vi "Additional_Post_Process_SJ_Data.vi"() -> ()   [LabVIEW 2012]
uses:
  Process_States.ctl
  Controls/SJ_Test_Matrix.ctl
  Controls/Analysis_info_cluster.ctl
  Controls/Inst_type.ctl
  Controls/Instrument_Array.ctl
  <vilib>/gmath/NumericalOptimization/stopping criteria.ctl
  <vilib>/Analysis/baseanly.llb/Scale 1D.vi
  <vilib>/Analysis/NI_AALBase.lvlib
  <vilib>/gmath/NI_Gmath.lvlib
panel:
  out "New Filename":path
  out "Prog bar":sgl(slide) scale=0.0..1.0
  out "Message":string
  in  "Max Iterations":i32=3000
  in  "Tolerance":dbl=0.0001
  in  "Raw Data Folder":path=path "F:/Enflo_Data_Local/2011/Aero_Tunnel/nick_martin/Raw_Measurements/11-2011/New_SJ_TestI_xls"
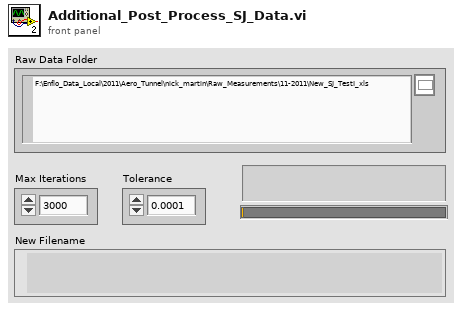
[diagram p1: front panel]
types:
  T1 = typedef "Process_States.ctl" = enum16{"Load Data", "Fit Parabolas", "Save Data"}
  T2 = typedef "SJ_Test_Matrix.ctl" = cluster{"Channel Data":cluster{"Amplitude (V)":dbl, "Phase Average":dbl[][], "Phase Angle":dbl[], "Frequency (Hz)":dbl, "AS Freq":dbl, "Zero":dbl, "Analysis info cluster":T3, "Radius":dbl[], "Beta":dbl, "Phi":dbl, "|Qd|":dbl, "Qd":dbl[]}[]}
  T3 = typedef "Analysis_info_cluster.ctl" = cluster{"Colour":u32, "Inst type":T4, "Inst name":string, "Symbol":string, "Code name":string, "Extra Info":string, "Inst Array":T5, "Extra Titles":string[], "Extra Values":string[], "U":dbl, "u^2":dbl, "u^3":dbl, "u^4":dbl, "Skew_u":dbl, "Kurt_u":dbl, "Sd Error in Mean":dbl, "% u'/U":dbl, "X":dbl, "Y":dbl, "Z":dbl, "Timescale integral to 25%":dbl, "Sd Error in Variance":dbl, "Calib File":path, "Calib Constants":dbl[], "Output Position":bool, "Full Stats":bool, "Av Sampling Rate":dbl, "Av No of Samples":dbl, "Total Meas Time (s)":dbl, "ADAM Ch Name":string}
  T4 = typedef "Inst_type.ctl" = enum16{"Propeller anemometer", "Raw voltage", "Pressure Transducer", "Pitot-static tube", "Preston tube", "Hot wire", "Cross wire 1", "Cross wire 2", "Generic Linear", "Generic Polynomial", "Generic BackPoly", "Fast FID", "Thermocouple", "Cold wire", "Pulsed Wire", "LDA Vel", "LDA Tran time", "LDA Arr time"}
  T5 = typedef "Instrument_Array.ctl" = enum16{"PWA", "LDA", "Analogue"}
  T6 = typedef "NI_Gmath.lvlib/stopping criteria.ctl" = cluster{"function tolerance":dbl, "parameter tolerance":dbl, "max iterations":i32, "max function calls":i32, "gradient tolerance":dbl, "max time (sec)":dbl}
  T7 = cluster{"Amplitude (V)":dbl, "Phase Average":dbl[][], "Phase Angle":dbl[], "Frequency (Hz)":dbl, "AS Freq":dbl, "Zero":dbl, "Analysis info cluster":T3, "Radius":dbl[], "Beta":dbl, "Phi":dbl, "|Qd|":dbl, "Qd":dbl[]}[]
  T8 = cluster{"Amplitude (V)":dbl, "Phase Average":dbl[][], "Phase Angle":dbl[], "Frequency (Hz)":dbl, "AS Freq":dbl, "Zero":dbl, "Analysis info cluster":T3, "Radius":dbl[], "Beta":dbl, "Phi":dbl, "|Qd|":dbl, "Qd":dbl[]}
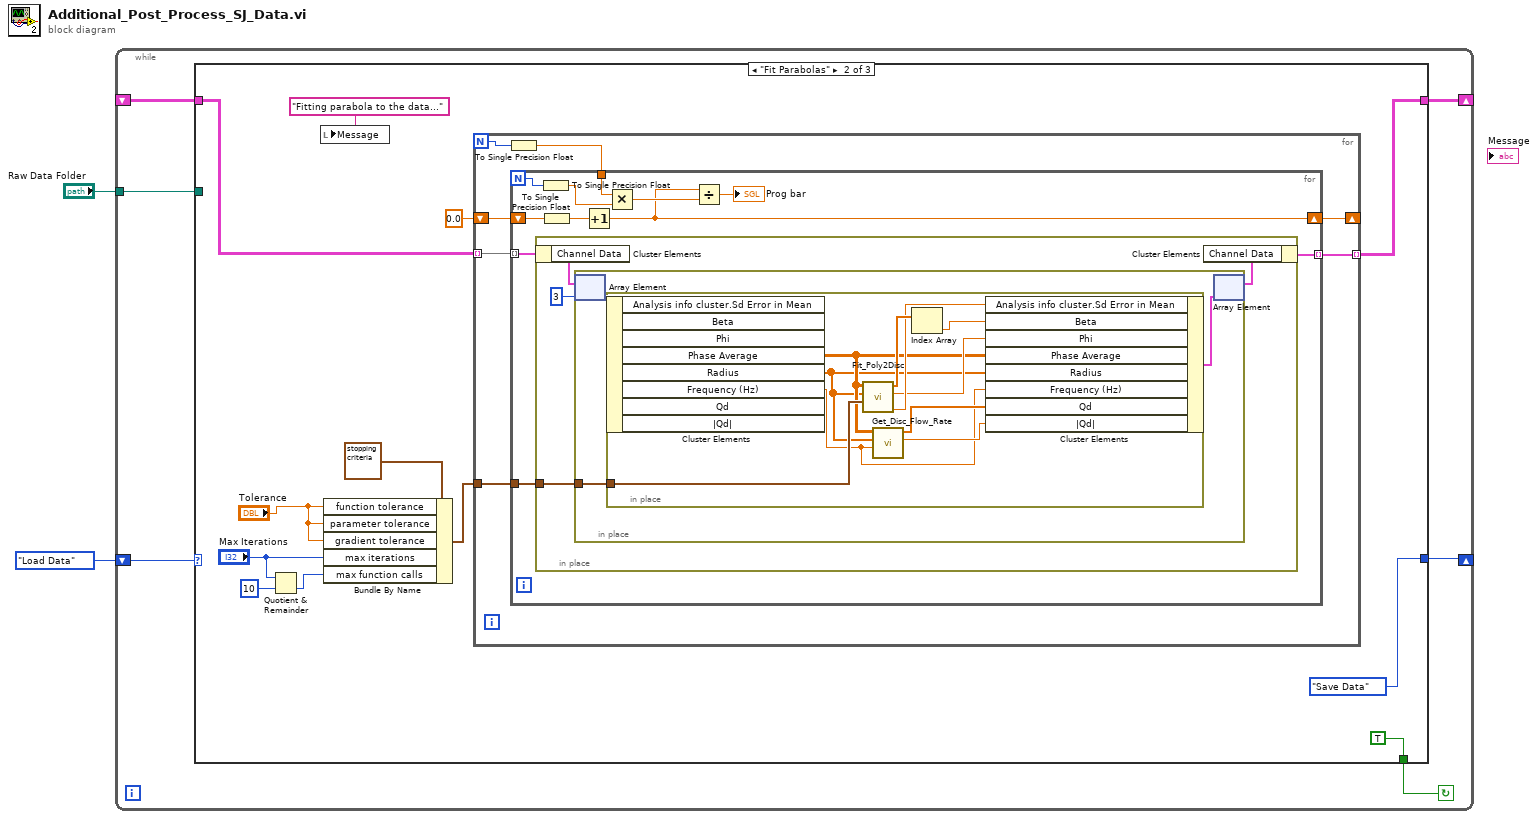
[diagram p0: block diagram]
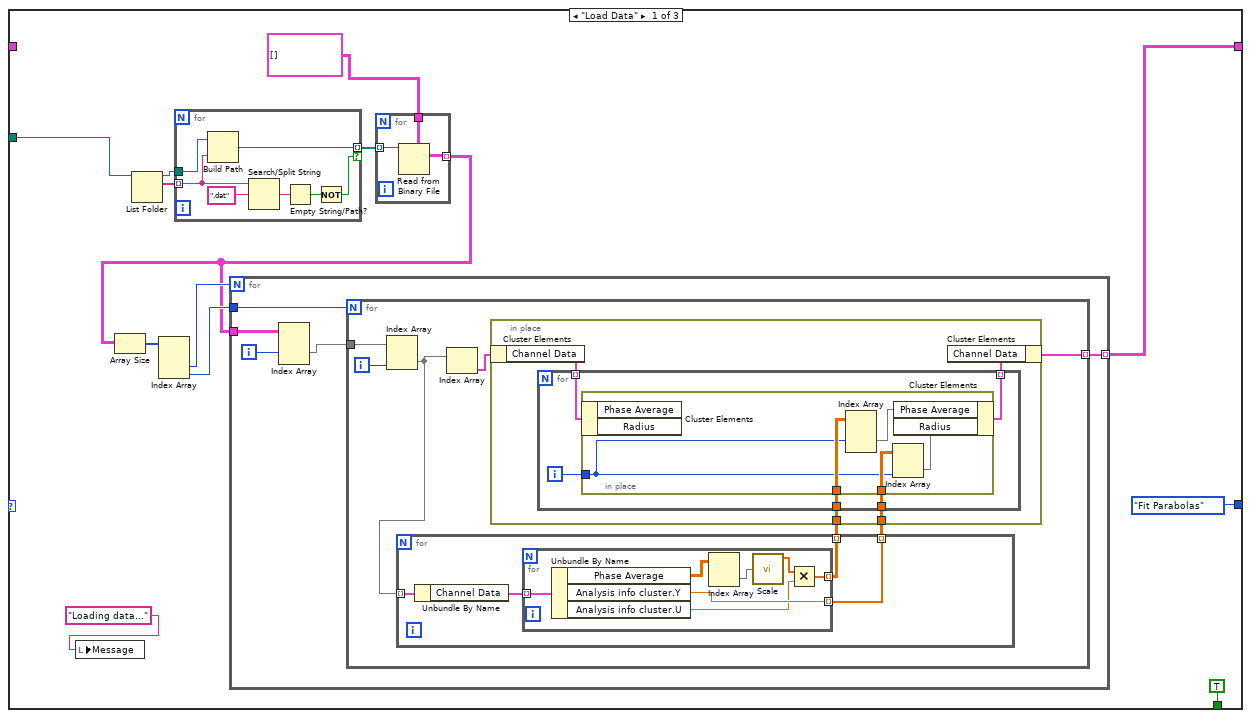
[diagram p2: hidden frame]
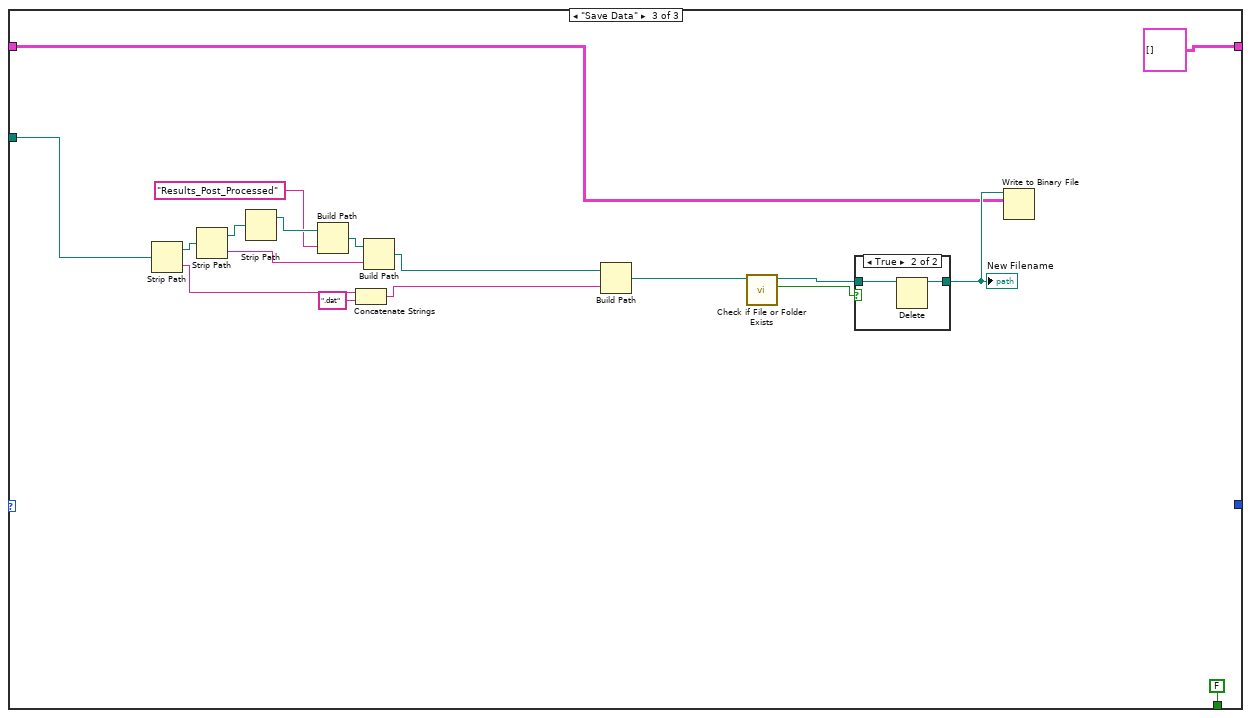
[diagram p3: hidden frame]
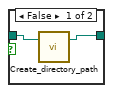
[diagram p4: hidden frame]
diagram:
  n1 = while {
    shift-right: [w7] -> _
    shift-left: _ -> [w6]
    shift-right: [w5] -> _
    shift-left: Process_States."Load Data" -> [w8]
    tunnel: "Raw Data Folder" -> [w3]
    stop <- w4 continue-if-true
    n2 = case shown="\"Fit Parabolas\"" w8 {
      tunnel: [w18 w71 T2[][] []] -> w7
      tunnel: w6 -> [_ w72 w116]
      tunnel: [Process_States."Fit Parabolas" ("Enum") Process_States."Save Data" ("Enum") _] -> w5
      tunnel: [TRUE TRUE FALSE] -> w4
      tunnel: w3 -> [w10 _ w120]
      frame "Load Data" {
        n3 = local write "Message"("Loading data..." ("Message")) -> ()
        n4 = List Folder(path=w10) -> (path out=w13:path, filenames=w12:string[])  [unwired: 3 in, 2 out]
        n5 = for {
          tunnel: w12 -> [w26] mode=indexing
          tunnel: [w25] -> w14 mode=indexing if=w29
          tunnel: w13 -> [w27]
          n6 = Build Path(base path=w27, name or relative path=w26) -> (appended path=w25:path)
          n7 = Search/Split String(string=w26, search string/char (-)=".dat" ("regular expression")) -> (match + rest of string=w28:string)  [unwired: 1 in, 2 out]
          n8 = Empty String/Path?(string/path=w28) -> (empty?=w30:bool)
          n9 = Not(x=w30) -> (.not. x?=w29:bool)
        }
        n10 = for {
          tunnel: w14 -> [w24] mode=indexing
          tunnel: T2[][] [] -> [w23]
          tunnel: [w22] -> w11 mode=indexing
          n11 = Read from Binary File(5:w23, 11:w24) -> (2:w22:T2[][])  [unwired: 4 in, 3 out]
        }
        n12 = Array Size(array=w11) -> (size(s)=w21:i32[])
        n13 = Index Array(array=w21) -> (element #2=w20:i32, element #3=w19:i32)  [unwired: 3 in, 1 out]
        n14 = for {
          N: w20 -> [_]
          tunnel: w11 -> [w36]
          tunnel: w19 -> [w33]
          tunnel: [w32] -> w18 mode=indexing
          i -> [w35]
          n15 = Index Array(array=w36, index (dim 1)=w35) -> (element=w34:T2[][])  [unwired: 2 in]
          n16 = for {
            N: w33 -> [_]
            tunnel: w34 -> [w43]
            tunnel: [w37] -> w32 mode=indexing
            i -> [w42]
            n17 = Index Array(array=w43, index (col)=w42) -> (element=w41:T2[])  [unwired: 1 in]
            n18 = for {
              tunnel: w41 -> [w61] mode=indexing
              tunnel: [w58] -> w39 mode=indexing
              tunnel: [w59] -> w38 mode=indexing
              n19 = Unbundle By Name(w61) -> ("Channel Data"=w60:T7)
              n20 = for {
                tunnel: [w68] -> w59 mode=indexing
                tunnel: [w62] -> w58 mode=indexing
                tunnel: w60 -> [w65] mode=indexing
                n21 = Unbundle By Name(w65) -> ("Phase Average"=w67:dbl[][], "Analysis info cluster.Y"=w68:dbl, "Analysis info cluster.U"=w63:dbl)
                n22 = Index Array(array=w67) -> (element=w66:dbl[])  [unwired: 2 in]
                n23 = call-poly <vilib>:"Scale.vi"("X"=w66) -> ("Y=(X-offset)/scale"=w64:dbl[])  [unwired: 3 out]
                n24 = Multiply(x=w64, y=w63) -> (x*y=w62:dbl[])
              }
            }
            n25 = Index Array(array=w41) -> (element=w40:T2)  [unwired: 1 in]
            n26 = in-place {
              in-place-border: w39 -> [w47]
              in-place-border: w38 -> [w46]
              n27 = in-place-cluster #1(w40) -> ("Channel Data"=w44:T7)
              n28 = for {
                tunnel: w47 -> [w49]
                tunnel: w46 -> [w48]
                tunnel: [w52] -> w45 mode=indexing
                tunnel: w44 -> [w51] mode=indexing
                i -> [w50]
                n29 = in-place {
                  in-place-border: w49 -> [w57]
                  in-place-border: w50 -> [w54]
                  in-place-border: w48 -> [w55]
                  n30 = in-place-cluster #2(w51) -> ()  [unwired: 2 out]
                  n31 = Index Array(array=w57, index (dim 1)=w54) -> (element=w56:dbl[][])  [unwired: 2 in]
                  n32 = Index Array(array=w55, index (col)=w54) -> (element=w53:dbl[])  [unwired: 1 in]
                  n33 = in-place-cluster #2("Phase Average"=w56, "Radius"=w53) -> (w52:T8)
                }
              }
              n34 = in-place-cluster #1("Channel Data"=w45) -> (w37:T2)
            }
          }
        }
      }
      frame "Fit Parabolas" {
        n35 = Quotient & Remainder(x="Max Iterations", y=10) -> (floor(x/y)=w74:i32)  [unwired: 1 out]
        n36 = local write "Message"("Fitting parabola to the data..." ("Message")) -> ()
        n37 = Bundle By Name(cluster=T6 {"function tolerance"=0.001, "parameter tolerance"=0.001, "max iterations"=100, "max function calls"=1000, "gradient tolerance"=0.001, "max time (sec)"=-1.0} ("stopping criteria"), "function tolerance"="Tolerance", "parameter tolerance"="Tolerance", "gradient tolerance"="Tolerance", "max iterations"="Max Iterations", "max function calls"=w74) -> (w77:T6)
        n38 = for {
          N -> [w85]
          tunnel: w72 -> [w87] mode=indexing
          tunnel: w77 -> [w86]
          tunnel: [w84] -> w71 mode=indexing
          shift-right: [w81] -> _
          shift-left: sgl 0.0 ("single precision float") -> [w82]
          n39 = To Single Precision Float(number=w85) -> (single precision float=w83:sgl)
          n40 = for {
            N -> [w96]
            tunnel: w87 -> [w98] mode=indexing
            tunnel: w86 -> [w97]
            tunnel: w83 -> [w94]
            tunnel: [w92] -> w84 mode=indexing
            shift-right: [w88] -> w81
            shift-left: w82 -> [w90]
            n41 = in-place {
              in-place-border: w97 -> [w99]
              n42 = in-place-cluster #3(w98) -> ("Channel Data"=w102:T7)
              n43 = in-place {
                in-place-border: w99 -> [w104]
                n44 = in-place-array #4(w102, 3) -> (w105:T8)
                n45 = in-place {
                  in-place-border: w104 -> [w115]
                  n46 = in-place-cluster #5(w105) -> ("Phase Average"=w110:dbl[][], "Radius"=w109:dbl[], "Frequency (Hz)"=w106:dbl)  [unwired: 5 out]
                  n47 = call "Fit_Poly2Disc.vi"("stopping criteria"=w115, "Rc"=w109, "Xd(t,r)"=w110) -> ("f(minimum)"=w112:dbl, "Sine Phase"=w111:dbl, "P(x)"=w114:dbl[])  [unwired: 5 in, 1 out]
                  n48 = call "Get_Disc_Flow_Rate.vi"("Jet Frequency"=w106, "Radius"=w109, "Phase Average"=w110) -> ("|Qd|"=w107:dbl, "Qd(t)"=w108:dbl[])  [unwired: 6 in, 1 out]
                  n49 = Index Array(array=w114) -> (element=w113:dbl)  [unwired: 1 in]
                  n50 = in-place-cluster #5("Analysis info cluster.Sd Error in Mean"=w112, "Beta"=w113, "Phi"=w111, "Phase Average"=w110, "Radius"=w109, "Frequency (Hz)"=w106, "Qd"=w108, "|Qd|"=w107) -> (w103:T8)
                }
                n51 = in-place-array #4(w103) -> (w100:T7)  [unwired: 1 out]
              }
              n52 = in-place-cluster #3("Channel Data"=w100) -> (w92:T2)
            }
            n53 = To Single Precision Float(number=w96) -> (single precision float=w95:sgl)
            n54 = To Single Precision Float(number=w90) -> (single precision float=w89:sgl)
            n55 = Increment(x=w89) -> (x+1=w88:sgl)
            n56 = Multiply(x=w94, y=w95) -> (x*y=w93:sgl)
            n57 = Divide(x=w88, y=w93) -> (x/y=→"Prog bar":sgl)
          }
        }
      }
      frame "Save Data" {
        n58 = Strip Path(path=w120) -> (stripped path=w128:path, name=w119:string)
        n59 = Strip Path(path=w128) -> (stripped path=w127:path, name=w123:string)
        n60 = Strip Path(path=w127) -> (stripped path=w126:path)  [unwired: 1 out]
        n61 = Build Path(base path=w126, name or relative path="Results_Post_Processed") -> (appended path=w124:path)
        n62 = Concatenate Strings(w119, ".dat" ("string")) -> (w117:string)
        n63 = Build Path(base path=w124, name or relative path=w123) -> (appended path=w122:path)
        n64 = Build Path(base path=w122, name or relative path=w117) -> (appended path=w121:path)
        n65 = call <vilib>:"Check if File or Folder Exists.vi"("path"=w121) -> ("file or folder exists?"=w131:bool, "dup path"=w130:path)  [unwired: 8 in, 1 out]
        n66 = case shown="True" w131 {
          tunnel: w130 -> [w135 w137]
          tunnel: [w134 w136] -> w129
          frame False {
            n67 = call "Create_directory_path.vi"("Path name"=w135) -> ("Path name Out"=w134:path)  [unwired: 1 in, 1 out]
          }
          frame True {
            n68 = Delete(path (use dialog)=w137) -> (deleted path=w136:path)  [unwired: 4 in, 2 out]
          }
        }
        "New Filename" <- w129
        n69 = Write to Binary File(file (use dialog)=w129, data=w116) -> ()  [unwired: 4 in, 3 out]
      }
    }
  }
